vi "车牌识别.vi"() -> ()   [LabVIEW 2015]
uses:
  C:/Program Files/MVTec/HALCON-10.0/bin/dotnet35/hdevenginedotnet.dll
  Program Files/MVTec/HALCON-10.0/bin/dotnet35/hdevenginedotnet.dll
  C:/Program Files/MVTec/HALCON-10.0/bin/dotnet35/halcondotnet.dll
  Program Files/MVTec/HALCON-10.0/bin/dotnet35/halcondotnet.dll
panel:
  out "Image":T1(plugin-control)
  out "D 2":dbl
  out "D":dbl
  out "SArr":string[](array[string])
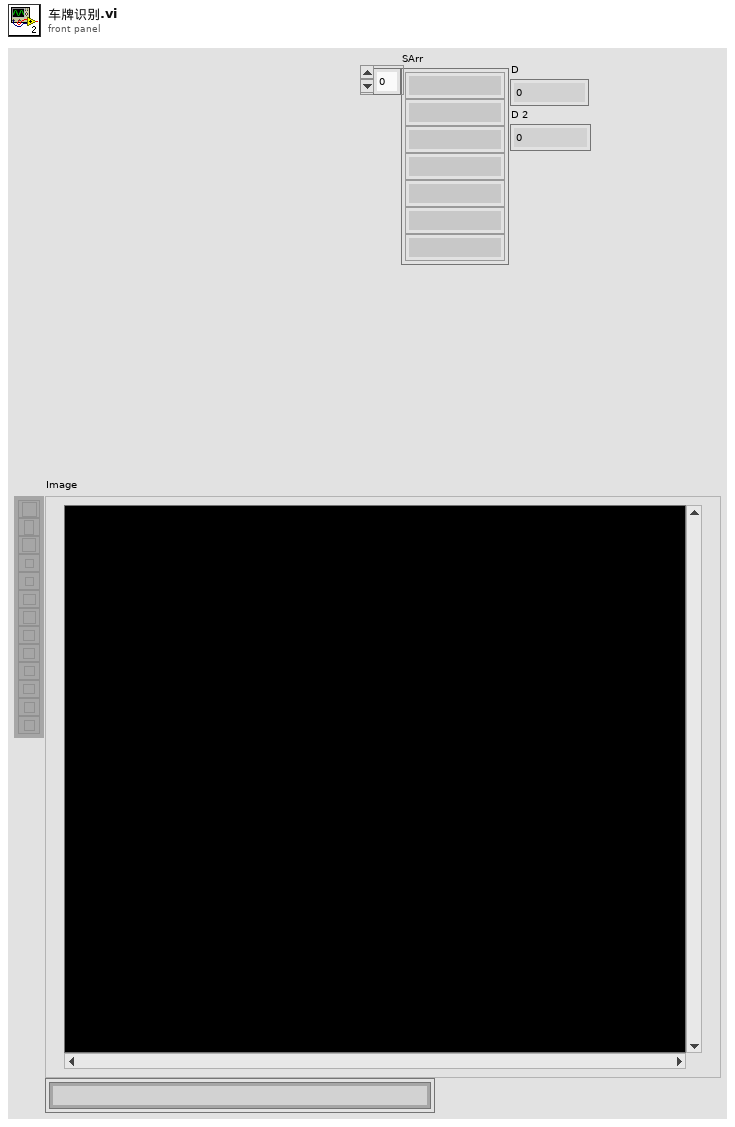
[diagram p1: front panel]
types:
  T1 = typedef "IMAQ Image.ctl" = refnum<image>
  T2 = typedef "Image Type" = u32
  T3 = cluster{"Desired Font (Application)":enum16{"User-specified Font", "Application Font", "System Font", "Dialog Font"}, "[User-specified Font]":cluster{"Font Name":string, "Size":i16, "Strikeout?":bool, "Italic?":bool, "Underline?":bool, "Outline?":bool, "Shadow?":bool, "Bold?":bool, "Rotation Angle":dbl}, "Horizontal Alignment":i16, "Vertical Alignment":i16}
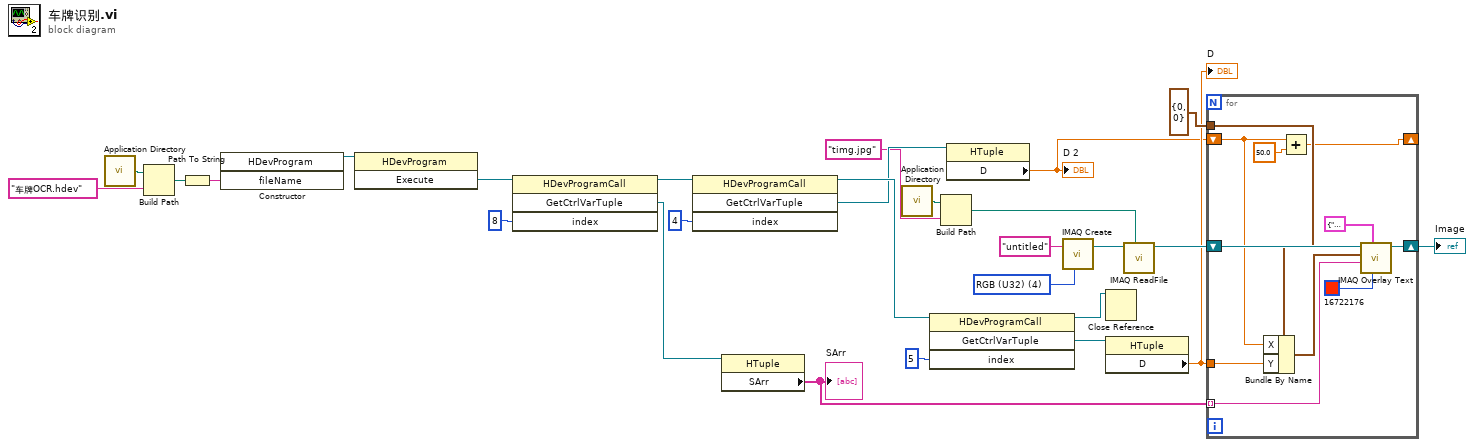
[diagram p0: block diagram]
diagram:
  w8 = T2 4 items=["Grayscale (U8)", "Grayscale (I16)", "Grayscale (SGL)", "Complex (CSG)", "RGB (U32)", "HSL (U32)", "RGB (U64)", "Grayscale (U16)"] ("Image Type")
  n1 = call <vilib>:"Application Directory.vi"() -> ("Application Directory"=w7:path)
  n2 = Build Path(base path=w7, name or relative path="车牌OCR.hdev") -> (appended path=w6:path)
  n3 = Path To String(path=w6) -> (string=w4:string)
  n4 = constructor class="HDevProgram"("fileName"=w4) -> (reference out=w25:refnum<k24>)  [unwired: 3 in, 3 out]
  n5 = invoke class="HDevProgram" method="Execute"(reference=w25) -> ("Execute"=w24:refnum<k24>)  [unwired: 2 in, 2 out]
  n6 = invoke class="HDevProgramCall" method="GetCtrlVarTuple"(reference=w24, "index"=8) -> (reference out=w23:refnum<k24>, "GetCtrlVarTuple"=w26:refnum<k24>)  [unwired: 2 in, 2 out]
  n7 = invoke class="HDevProgramCall" method="GetCtrlVarTuple"(reference=w23, "index"=4) -> (reference out=w20:refnum<k24>, "GetCtrlVarTuple"=w19:refnum<k24>)  [unwired: 2 in, 2 out]
  n8 = property on="属性节点" class="HTuple"(reference=w26) -> ("SArr"=w13:string[])  [unwired: 1 in, 2 out]
  "SArr" <- w13
  n9 = call <vilib>:"Application Directory.vi"() -> ("Application Directory"=w2:path)
  n10 = invoke class="HDevProgramCall" method="GetCtrlVarTuple"(reference=w20, "index"=5) -> (reference out=w17:refnum<k24>, "GetCtrlVarTuple"=w18:refnum<k24>)  [unwired: 2 in, 2 out]
  n11 = Build Path(base path=w2, name or relative path="timg.jpg") -> (appended path=w1:path)
  n12 = property on="属性节点" class="HTuple"(reference=w19) -> ("D"=w9:dbl)  [unwired: 1 in, 2 out]
  "D 2" <- w9
  n13 = call "IMAQ Create"("Image Name"="untitled", "Image Type"=w8) -> ("New Image"=w15:T1)  [unwired: 3 in, 1 out]
  n14 = Close Reference(reference=w17) -> ()  [unwired: 1 in, 1 out]
  n15 = property on="属性节点" class="HTuple"(reference=w18) -> ("D"=w10:dbl)  [unwired: 1 in, 2 out]
  "D" <- w10
  n16 = call "IMAQ ReadFile"("File Path"=w1, "Image"=w15) -> ("Image Out"=w14:T1)  [unwired: 5 in, 4 out]
  n17 = for {
    tunnel: w13 -> [w37] mode=indexing
    shift-right: [w36] -> w12
    shift-left: w14 -> [w38]
    tunnel: cluster{"X":i32, "Y":i32} {"X"=0, "Y"=0} ("Origin") -> [w33]
    tunnel: w10 -> [w32]
    shift-right: [w29] -> _
    shift-left: w9 -> [w30]
    n18 = Bundle By Name(cluster=w33, "X"=w30, "Y"=w32) -> (w31:cluster{"X":i32, "Y":i32})
    n19 = Add(x=w30, y=50.0) -> (x+y=w29:dbl)
    n20 = call "IMAQ Overlay Text"("Text Color (black)"=u32 16722176, "Font, Size & Style"=T3 {"Desired Font (Application)"=enum."Application Font", "[User-specified Font]"={"Font Name"="", "Size"=20, "Strikeout?"=FALSE, "Italic?"=FALSE, "Underline?"=FALSE, "Outline?"=FALSE, "Shadow?"=FALSE, "Bold?"=FALSE, "Rotation Angle"=0.0}, "Horizontal Alignment"=0, "Vertical Alignment"=0}, "String"=w37, "Origin"=w31, "Image"=w38) -> ("Image Out"=w36:T1)  [unwired: 5 in, 1 out]
  }
  "Image" <- w12
